vi "lvEtherbone.device_write.vi"(0 "eb_socket_ID":i32, 1 "eb_device_ID":i32, 2 "address":u32 format="%.0x", 3 "data":u32 format="%.0x", 5 "error in (no error)":errorcluster) -> (13 "eb_status":T1 items=["EB_SUCCESS"=1, "EB_OK"=0, "EB_FAIL"=-1, "EB_ADDRESS"=-2, "EB_WIDTH"=-3, "EB_OVERFLOW"=-4, "EB_ENDIAN"=-5, "EB_BUSY"=-6, "EB_TIMEOUT"=-7, "EB_OOM"=-8, "EB_ABI"=-9, "EB_SEGFAULT"=-10], 14 "eb_socket_ID out":i32, 15 "eb_device_ID out":i32, 19 "error out":errorcluster)   [LabVIEW 2012, in "lvEtherbone.lvlib"]
doc: "/* Convenience methods which create single-operation cycles.\n * Equivalent to: eb_cycle_open, eb_cycle_{read,write}, eb_cycle_close.\n */\n\n\nEB_PUBLIC eb_status_t eb_device_write(eb_device_t device,\n eb_address_t address,\n eb_format_t format,\n eb_data_t data,\n eb_user_data_t user_data,\n eb_callback_t cb);"
uses:
  lvEtherbone.lvlib
  lvEtherbone.lveb_status_t.ctl
  libetherbone.so
panel:
  in  "eb_status_t":T1 items=["EB_SUCCESS"=1, "EB_OK"=0, "EB_FAIL"=-1, "EB_ADDRESS"=-2, "EB_WIDTH"=-3, "EB_OVERFLOW"=-4, "EB_ENDIAN"=-5, "EB_BUSY"=-6, "EB_TIMEOUT"=-7, "EB_OOM"=-8, "EB_ABI"=-9, "EB_SEGFAULT"=-10]
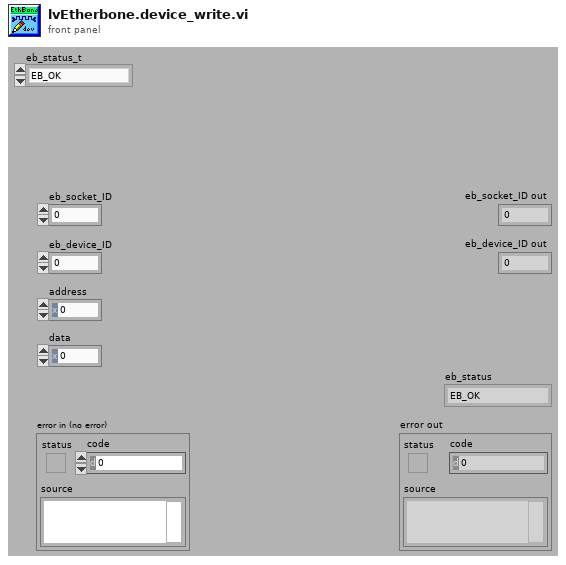
[diagram p1: front panel]
types:
  T1 = typedef "lvEtherbone.lvlib/lvEtherbone.lveb_status_t.ctl" = i32
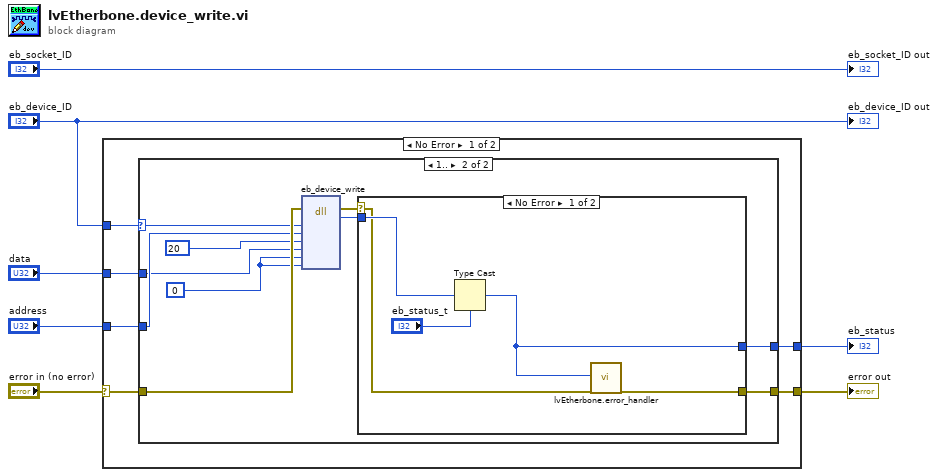
[diagram p0: block diagram]
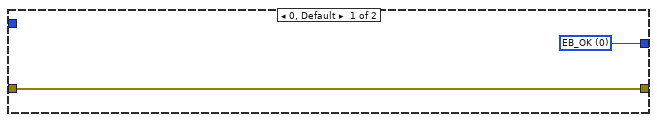
[diagram p2: hidden frame]
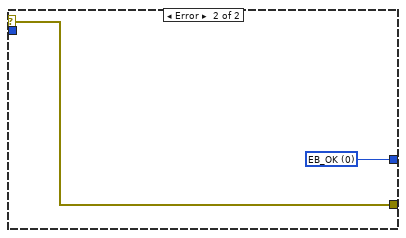
[diagram p3: hidden frame]
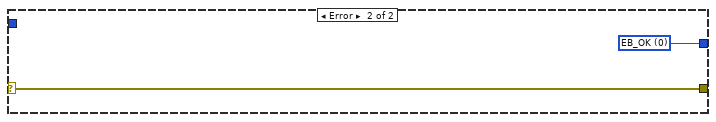
[diagram p4: hidden frame]
diagram:
  n1 = case shown="No Error" "error in (no error)" {
    selector: "error in (no error)" -> [w13 w34]
    tunnel: [w12 w34] -> w6
    tunnel: "address" -> [w10 _]
    tunnel: "eb_device_ID" -> [w9 _]
    tunnel: [w11 w33] -> w4
    tunnel: "data" -> [w8 _]
    frame No Error {
      n2 = case shown="1.." w9 {
        selector: w9 -> [_ w19]
        tunnel: w13 -> [w14 w23]
        tunnel: [w14 w22] -> w12
        tunnel: [w15 w21] -> w11
        tunnel: w10 -> [_ w20]
        tunnel: w8 -> [_ w17]
        frame 0, Default {
          w15 = T1 0 items=["EB_SUCCESS"=1, "EB_OK"=0, "EB_FAIL"=-1, "EB_ADDRESS"=-2, "EB_WIDTH"=-3, "EB_OVERFLOW"=-4, "EB_ENDIAN"=-5, "EB_BUSY"=-6, "EB_TIMEOUT"=-7, "EB_OOM"=-8, "EB_ABI"=-9, "EB_SEGFAULT"=-10] ("eb_status_t")
        }
        frame 1.. {
          w16 = u32 0 ("user_data")
          n3 = dll-call lib="libetherbone.so" fn="eb_device_write"(error in=w23, "device"=w19, "address"=w20, "format"=u8 20, "data"=w17, "user_data"=w16, "cb"=w16) -> (error out=w24:errorcluster, "eb_status"=w25:i32)  [unwired: 8 in, 1 out]
          n4 = case shown="No Error" w24 {
            selector: w24 -> [w27 w32]
            tunnel: w25 -> [w30 _]
            tunnel: [w28 w31] -> w21
            tunnel: [w26 w32] -> w22
            frame No Error {
              n5 = Type Cast(type="eb_status_t", x=w30) -> (*(type *) &x=w28:T1)
              n6 = call "lvEtherbone.error_handler.vi"("eb_status"=w28, "error in"=w27) -> ("error out"=w26:errorcluster)  [unwired: 17 in]
            }
            frame Error {
              w31 = T1 0 items=["EB_SUCCESS"=1, "EB_OK"=0, "EB_FAIL"=-1, "EB_ADDRESS"=-2, "EB_WIDTH"=-3, "EB_OVERFLOW"=-4, "EB_ENDIAN"=-5, "EB_BUSY"=-6, "EB_TIMEOUT"=-7, "EB_OOM"=-8, "EB_ABI"=-9, "EB_SEGFAULT"=-10] ("eb_status_t")
            }
          }
        }
      }
    }
    frame Error {
      w33 = T1 0 items=["EB_SUCCESS"=1, "EB_OK"=0, "EB_FAIL"=-1, "EB_ADDRESS"=-2, "EB_WIDTH"=-3, "EB_OVERFLOW"=-4, "EB_ENDIAN"=-5, "EB_BUSY"=-6, "EB_TIMEOUT"=-7, "EB_OOM"=-8, "EB_ABI"=-9, "EB_SEGFAULT"=-10] ("eb_status_t")
    }
  }
  "error out" <- w6
  "eb_status" <- w4
  "eb_socket_ID out" <- "eb_socket_ID"
  "eb_device_ID out" <- "eb_device_ID"
